vi "Initialize Tree List.vi"(8 "error in (no error)":errorcluster, 10 "List in":T1[](array[typedef]), 11 "TreeControl in":refnum<vi>) -> (0 "error out":errorcluster, 3 "TreeControl out":refnum<vi>)   [LabVIEW 2015, in "Shared Variable Custom Device.lvlib"]
uses:
  Shared Variable Custom Device.lvlib
  Tree Data.ctl
  <vilib>/Utility/VariantDataType/Type.ctl
  <vilib>/Utility/VariantDataType/VariantType.lvlib
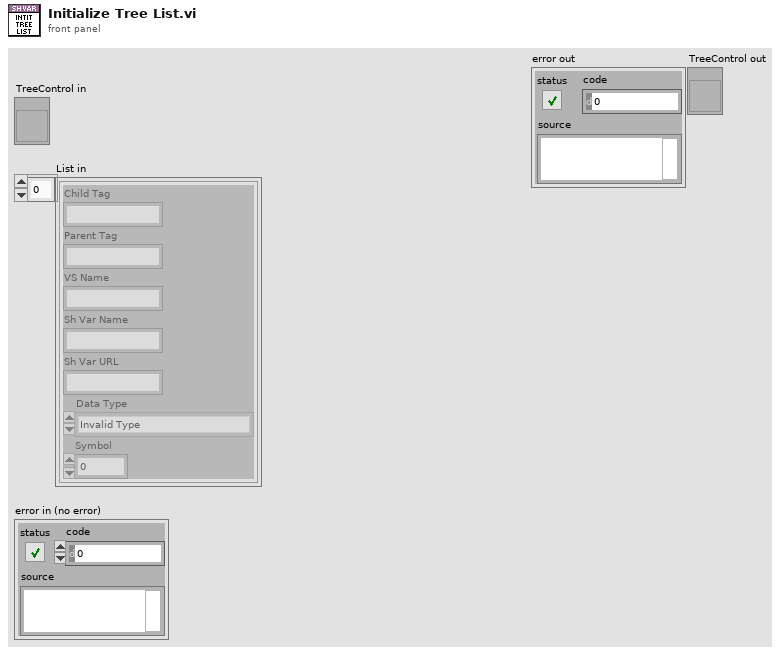
[diagram p1: front panel]
types:
  T1 = typedef "Shared Variable Custom Device.lvlib/Tree Data.ctl" = cluster{"Child Tag":string, "Parent Tag":string, "VS Name":string, "Sh Var Name":string, "Sh Var URL":string, "Data Type":T2, "Symbol":i32}
  T2 = typedef "VariantType.lvlib/Type.ctl" = enum8{"Invalid Type", "Void", "I8", "I16", "I32", "I64", "U8", "U16", "U32", "U64", "Single Float", "Double Float", "Extended Float", "Single Complex", "Double Complex", "Extended Complex", "Enum U8", "Enum U16", "Enum U32", "Enum U64", "Single Float With Unit", "Double Float With Unit", "Extended Float With Unit", "Single Complex with Unit", "Double Complex with Unit", "Extended Complex with Unit", "Boolean", "String", "Path", "Picture", "Tag", "Array", "Cluster", "Variant", "LV Variant", "Waveform", "Timestamp", "Digital Waveform", "Digital Data", "ExpressData", "Refnum", "External Data", "VI", "Poly VI", "LabVIEW Class Instance", "Fixed Point"}
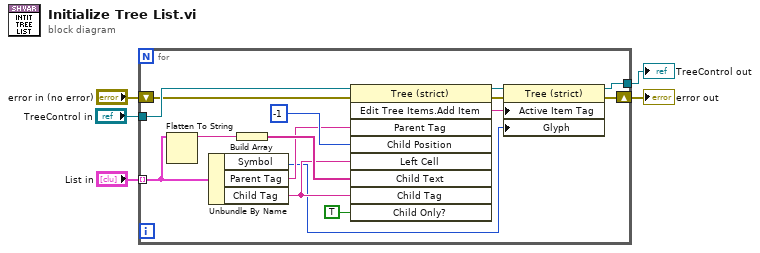
[diagram p0: block diagram]
diagram:
  n1 = for {
    tunnel: "TreeControl in" -> [w9]
    tunnel: "List in" -> [w13] mode=indexing
    shift-right: [w7] -> w2
    shift-left: "error in (no error)" -> [w8]
    tunnel: [w6] -> w1
    n2 = Flatten To String(anything=w13) -> (data string=w19:string)  [unwired: 3 in, 2 out]
    n3 = Unbundle By Name(w13) -> ("Symbol"=w10:i32, "Parent Tag"=w12:string, "Child Tag"=w11:string)
    n4 = Build Array(w19) -> (w20:string[])
    n5 = invoke class="Tree (strict)" method="Edit Tree Items.Add Item"(reference=w9, error in=w8, "Parent Tag"=w12, "Child Position"=-1, "Left Cell"=w11, "Child Text"=w20, "Child Tag"=w11, "Child Only?"=TRUE) -> (reference out=w16:refnum<vi>, error out=w17:errorcluster, "Edit Tree Items:Add Item"=w15:string)  [unwired: 1 in, 6 out]
    n6 = property class="Tree (strict)"(reference=w16, error in=w17, "Active Item Tag"=w15, "Glyph"=w10) -> (reference out=w6:refnum<vi>, error out=w7:errorcluster)
  }
  "error out" <- w2
  "TreeControl out" <- w1
